vi "Configure Common.vi"(0 "Instrument Handle In":refnum<k21>, 1 "Selector String":string, 5 "Common Configuration":T1={"Measurement Interval (s)"=0.0001, "Signal Type"=0, "DUT Average Input Power (dBm)"=-15.0, "Synchronization Method"=1} {"Synchronization Method" items=["False", "True"]; "DUT Average Input Power (dBm)" format="%.2f"; "Signal Type" items=["Modulated", "Tones"]; "Measurement Interval (s)" format="%#.2p"}, 7 "Waveform":T2={"Waveform Name"="Wfm", "Waveform"={"x0"=0.0, "dx"=0.0, "y"=[]}, "Signal Bandwidth (Hz)"=0.0, "PAPR (dB)"=0.0, "Burst Length (s)"=0.0, "Sample Rate"=0.0, "Burst Start Locations"=[], "Burst Stop Locations"=[], "Idle Duration Present?"=FALSE, "Runtime Scaling"=0.0, "Script"=""} {"Runtime Scaling" format="%#_6p"; "Sample Rate" format="%#_6p"; "Burst Length (s)" format="%#_6p"; "PAPR (dB)" format="%.2f"; "Signal Bandwidth (Hz)" format="%#_6p"; "Waveform"."y" format="%.2f"; "Waveform"."dx" format="%^.2e"; "Waveform"."x0" format="%^.2e"}, 11 "error in (no error)":errorcluster) -> (4 "Instrument Handle Out":refnum<k21>, 15 "error out":errorcluster)   [LabVIEW 2016, in "RFmxDPD.lvlib"]
uses:
  RFmxDPD.lvlib
  SG/Typedefs/Waveform.ctl
  Typedefs/Common Configuration.ctl
  <vilib>/RFmx/SpecAn/mx/RFmxSpecAn.llb/RFmxSpecAn Select Measurement (Single).vi
  SG/SG.lvlib
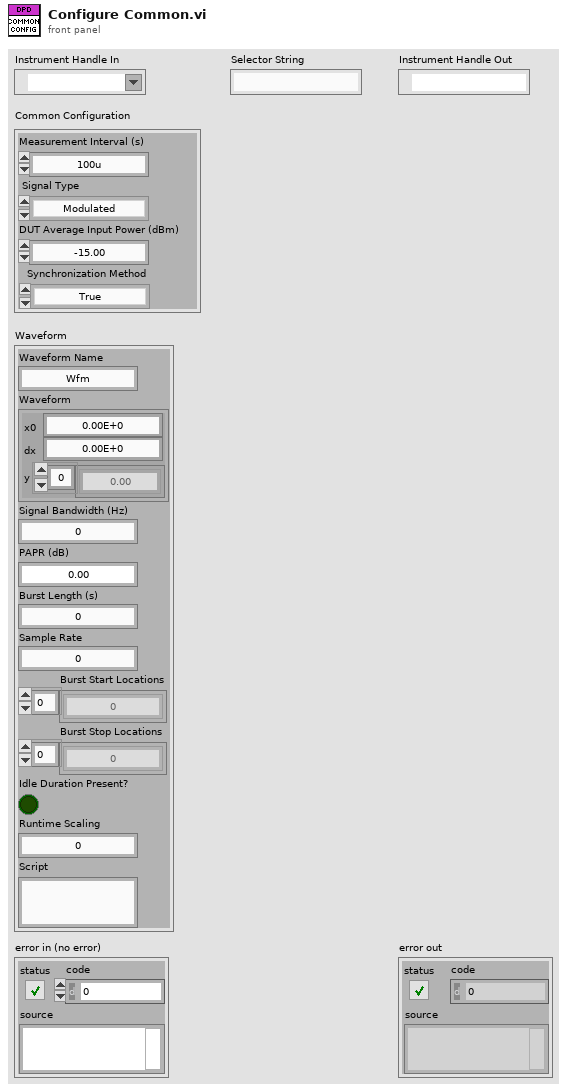
[diagram p1: front panel]
types:
  T1 = typedef "RFmxDPD.lvlib/Common Configuration.ctl" = cluster{"Measurement Interval (s)":dbl, "Signal Type":i32, "DUT Average Input Power (dBm)":dbl, "Synchronization Method":i32}
  T2 = typedef "SG.lvlib/Waveform.ctl" = cluster{"Waveform Name":string, "Waveform":cluster{"x0":dbl, "dx":dbl, "y":csg[]}, "Signal Bandwidth (Hz)":dbl, "PAPR (dB)":dbl, "Burst Length (s)":dbl, "Sample Rate":dbl, "Burst Start Locations":i32[], "Burst Stop Locations":i32[], "Idle Duration Present?":bool, "Runtime Scaling":dbl, "Script":string}
  T3 = enum16{"ACP", "CCDF", "CHP", "FCnt", "Harmonics", "OBW", "SEM", "Spectrum", "Spur", "TXP", "AMPM", "DPD", "IQ", "IM", "NF", "PhaseNoise"}
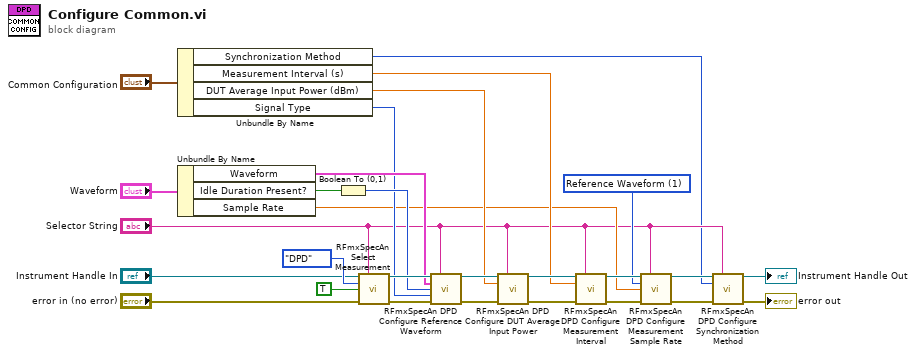
[diagram p0: block diagram]
diagram:
  w8 = 1 items=["User", "Reference Waveform"] ("Sample Rate Mode")
  n1 = Unbundle By Name("Common Configuration") -> ("Synchronization Method"=w3:i32, "Measurement Interval (s)"=w10:dbl, "DUT Average Input Power (dBm)"=w11:dbl, "Signal Type"=w12:i32)
  n2 = Unbundle By Name("Waveform") -> ("Waveform"=w16:cluster{"x0":dbl, "dx":dbl, "y":csg[]}, "Idle Duration Present?"=w15:bool, "Sample Rate"=w7:dbl)
  n3 = Boolean To (0,1)(Boolean=w15) -> (0, 1=w14:i16)
  n4 = call-poly <vilib>:"RFmxSpecAn Select Measurement.vi"("Instrument Handle In"="Instrument Handle In", "Selector String"="Selector String", "Measurement"=T3."DPD", "Enable All Traces"=TRUE, "error in (no error)"="error in (no error)") -> ("Instrument Handle Out"=w25:refnum<k21>, "error out"=w24:errorcluster)  [unwired: 9 in]
  n5 = call <vilib>:"RFmxSpecAn DPD Configure Reference Waveform.vi"("Instrument Handle In"=w25, "Selector String"="Selector String", "Reference Waveform"=w16, "Idle Duration Present"=w14, "Signal Type"=w12, "error in (no error)"=w24) -> ("Instrument Handle Out"=w23:refnum<k21>, "error out"=w22:errorcluster)  [unwired: 8 in]
  n6 = call <vilib>:"RFmxSpecAn DPD Configure DUT Average Input Power.vi"("Instrument Handle In"=w23, "Selector String"="Selector String", "DUT Average Input Power (dBm)"=w11, "error in (no error)"=w22) -> ("Instrument Handle Out"=w21:refnum<k21>, "error out"=w20:errorcluster)  [unwired: 10 in]
  n7 = call <vilib>:"RFmxSpecAn DPD Configure Measurement Interval.vi"("Instrument Handle In"=w21, "Selector String"="Selector String", "Measurement Interval (s)"=w10, "error in (no error)"=w20) -> ("Instrument Handle Out"=w19:refnum<k21>, "error out"=w18:errorcluster)  [unwired: 10 in]
  n8 = call <vilib>:"RFmxSpecAn DPD Configure Measurement Sample Rate.vi"("Instrument Handle In"=w19, "Selector String"="Selector String", "Sample Rate Mode"=w8, "Sample Rate (S/s)"=w7, "error in (no error)"=w18) -> ("Instrument Handle Out"=w6:refnum<k21>, "error out"=w5:errorcluster)  [unwired: 9 in]
  n9 = call <vilib>:"RFmxSpecAn DPD Configure Synchronization Method.vi"("Instrument Handle In"=w6, "Selector String"="Selector String", "Synchronization Method"=w3, "error in (no error)"=w5) -> ("Instrument Handle Out"=→"Instrument Handle Out":refnum<k21>, "error out"=→"error out":errorcluster)  [unwired: 10 in]
